vi "High_Voltage_Power_Supply_API.vi"(0 "COM Port In":refnum<visa-resource-name>, 2 "Control Mode (T = CV, F = CC)":bool=TRUE, 3 "CH1 ON/OFF (T = ON)":bool, 4 "CH2 ON/OFF (T = ON)":bool, 5 "MEASURE (T = measure)":bool, 6 "STOP (T = stop)":bool, 7 "error in (no error)":errorcluster, 10 "CH1 VOLTAGE SET (-2000...0 V)":i16 min=-2000 max=0 step=100, 11 "CH2 VOLTAGE SET (0...+2000 V)":i16 min=0 max=2000 step=100, 12 "CH1 CURRENT SET (0...5 mA)":dbl=5.0 min=0.0 max=5.0 step=0.1 format="%_4f", 13 "CH2 CURRENT SET (0...5 mA)":dbl=5.0 min=0.0 max=5.0 step=0.1 format="%_4f") -> (20 "COM Port Out":refnum<visa-resource-name>, 21 "Connection (T = active)":bool, 22 "Emergency Stop (T = active)":bool, 23 "CH1 VOLTAGE OUT (V)":i32, 24 "CH1 CURRENT OUT (mA)":dbl format="%#_4f", 25 "CH2 VOLTAGE OUT (V)":i32, 26 "CH2 CURRENT OUT (mA)":dbl format="%#_4f", 27 "error out":errorcluster)   [LabVIEW 2016]
doc: "This VI controls the High Voltage Power Supply.\n\nUsage: \n # Place this VI in a while loop for continuous operation\n\nExtra information:\n # 2 channels CH:\n * CH1 outputs -2000 to 0 V\n * CH2 outputs 0 to +2000 V\n * Both output 0 to 5 mA\n\n # Control Mode:\n * True = CV or Constant Voltage: \"VOLTAGE SET\" sets the output voltage \n and \"CURRENT SET\" sets the current limit\n * False = CC or Constant Current: \"CURRENT SET\" sets the output current \n and \"VOLTAGE SET\" sets the voltage limit\n\n # Connection (T = active)\n * Signals whether a connection is established\n\n # Emergency Stop (T = active)\n * Signals whether the emergency stop is on\n\n # Measure (T = measure):\n * True: Constant or pulse\n\n # Stop (T = stop)\n * True: Pulse\n * Resets the High Voltage Power Supply\n\nBachelor's thesis FIIW 3Ba EA-ICT 2017-2018:\n * Sven Baerten - sven.baerten@student.uhasselt.be\n * Wouter Falise - wouter.falise@student.uhasselt.be"
uses:
  High_Voltage_Power_Supply_API_States.ctl
  <vilib>/Instr/_visa.llb/VISA Configure Serial Port (Instr).vi
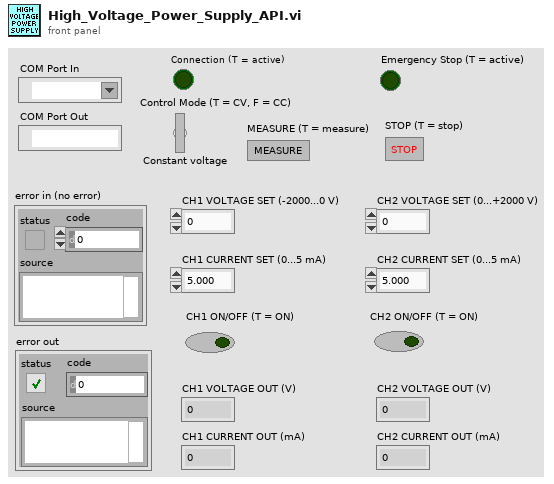
[diagram p1: front panel]
types:
  T1 = typedef "High_Voltage_Power_Supply_API_States.ctl" = enum16{"EMERGENCY_STOP", "NOT_SYNCHRONISED", "SYNCHRONISED"}
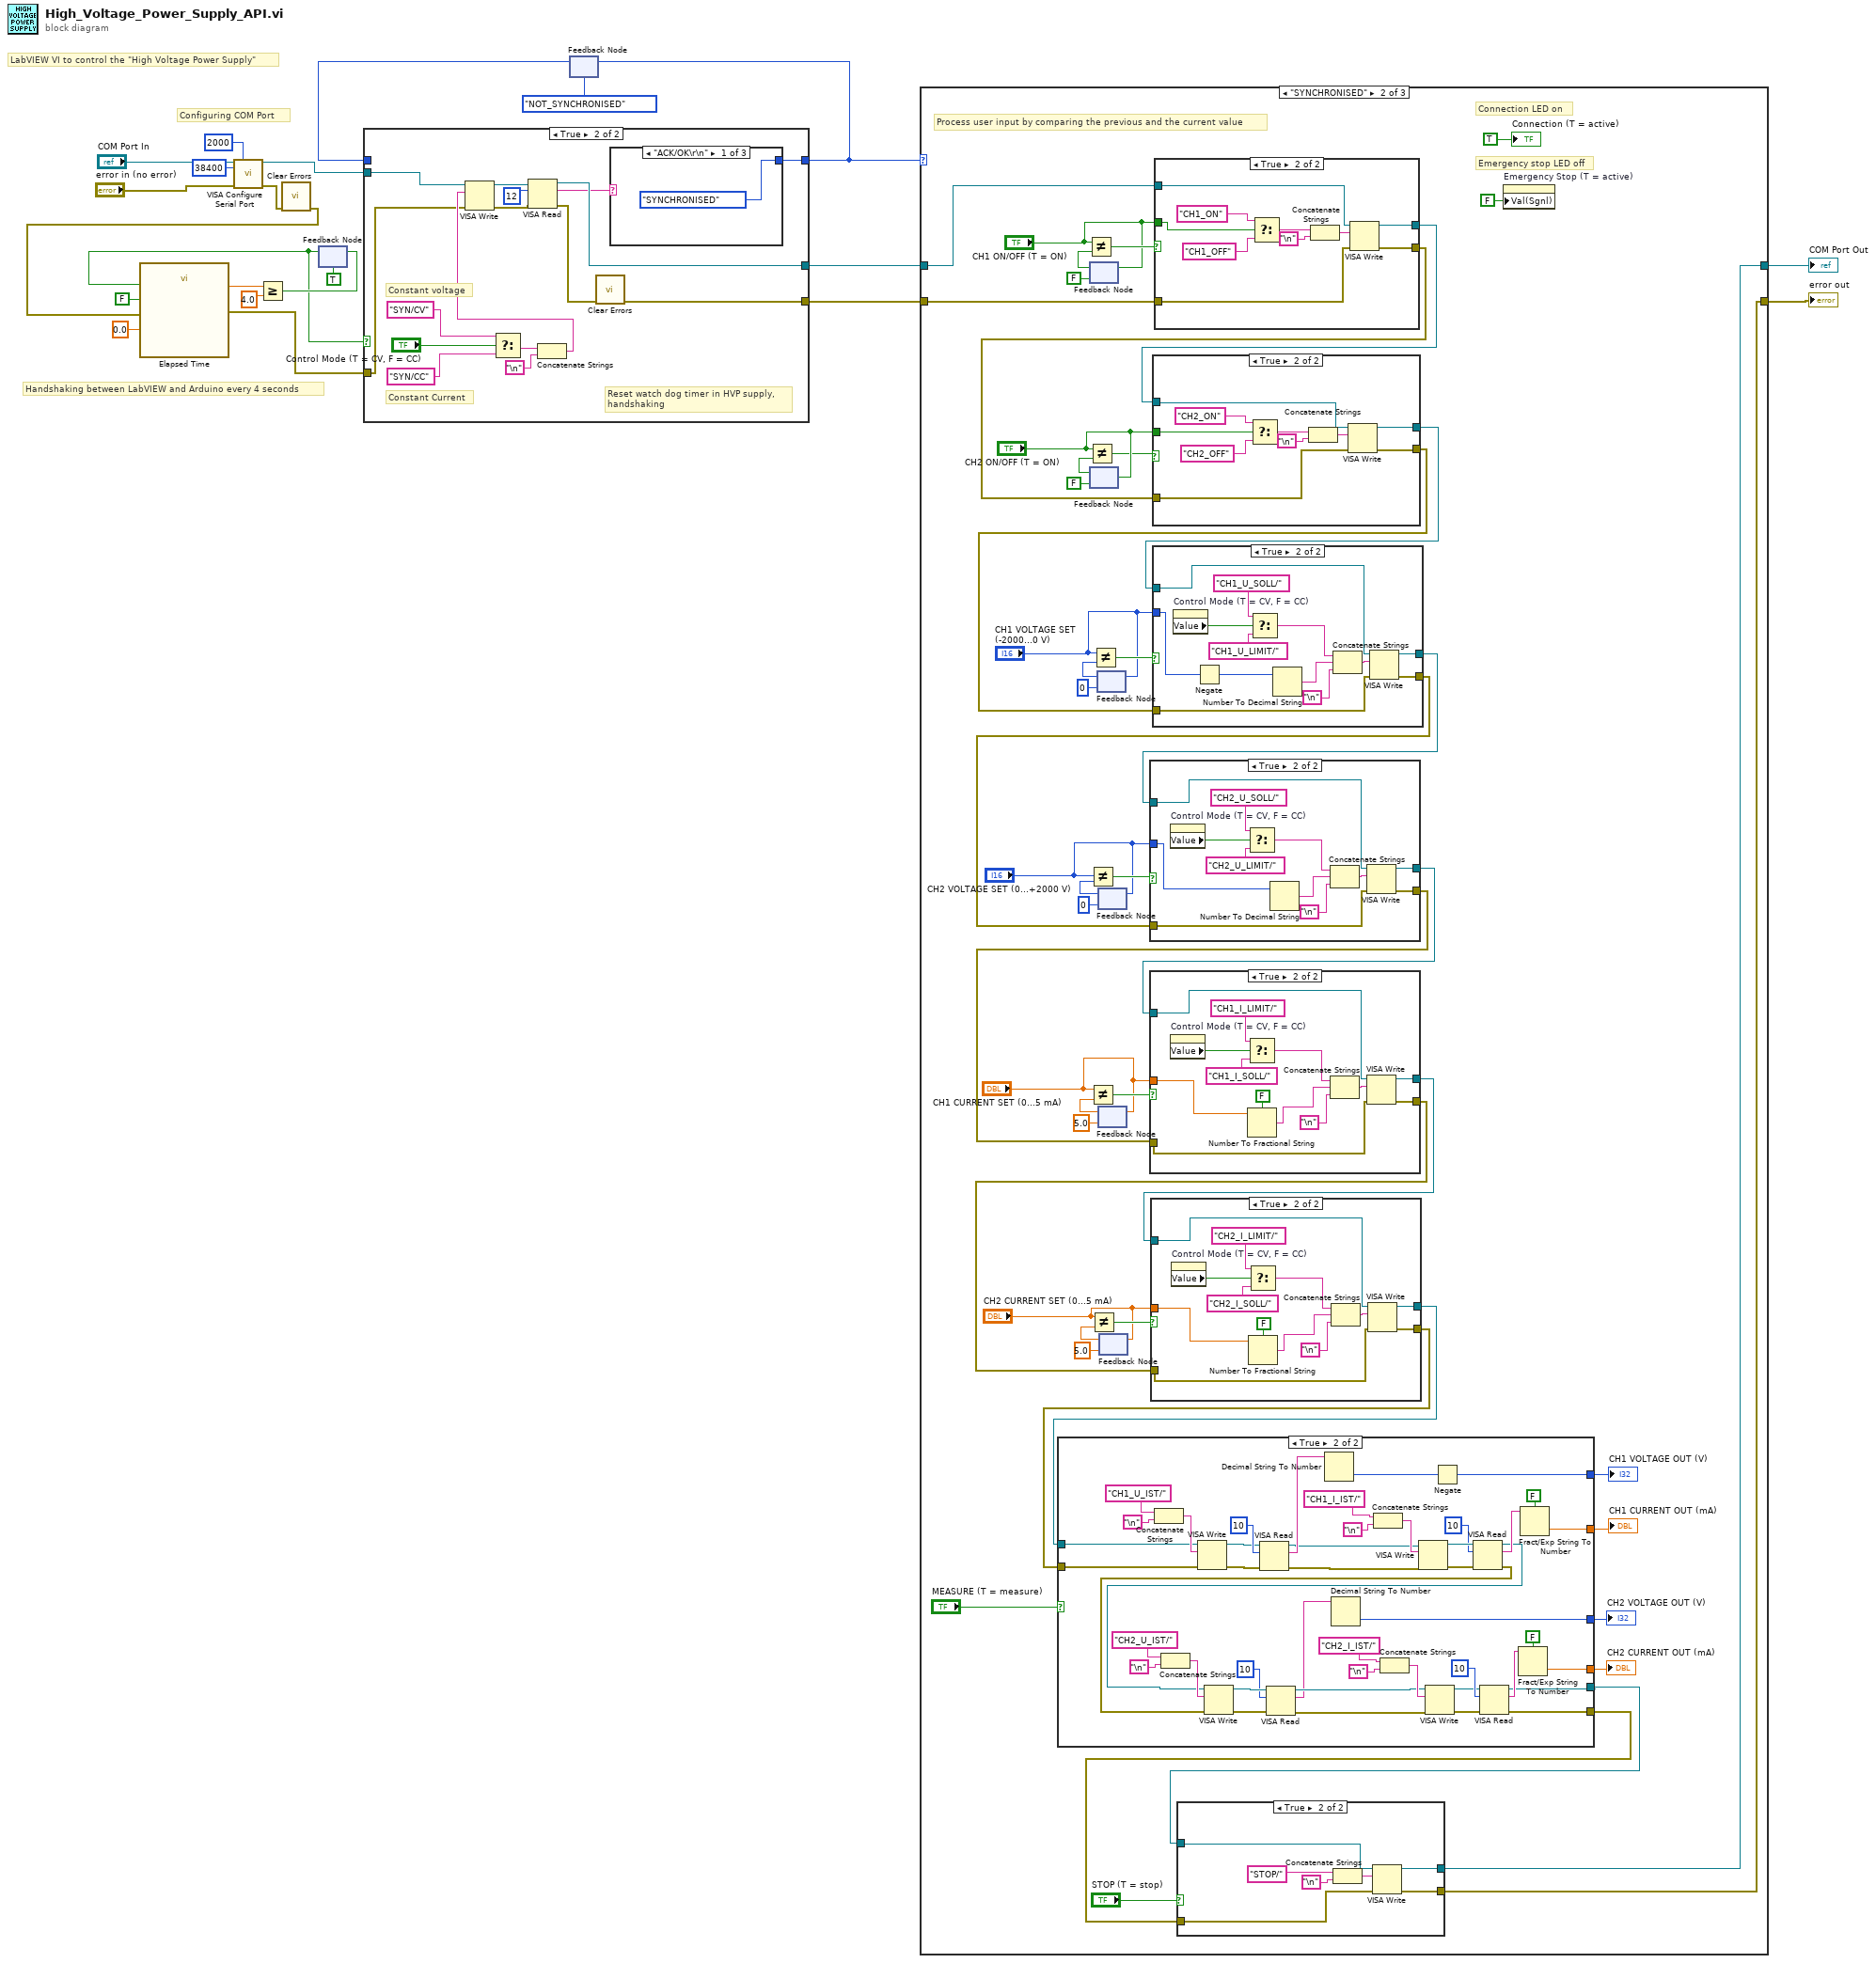
[diagram p0: block diagram]
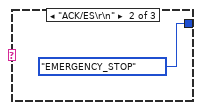
[diagram p3: hidden frame]
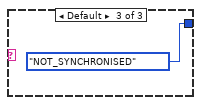
[diagram p4: hidden frame]
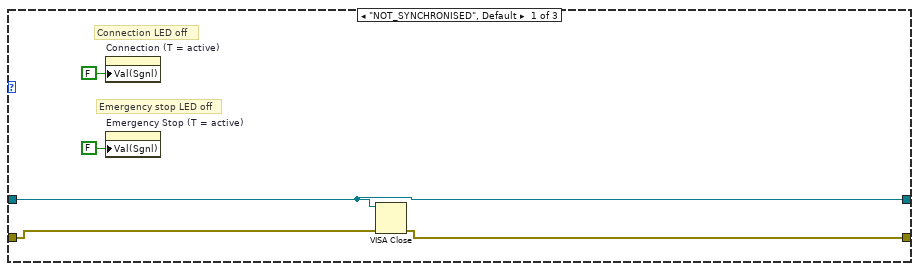
[diagram p5: hidden frame]
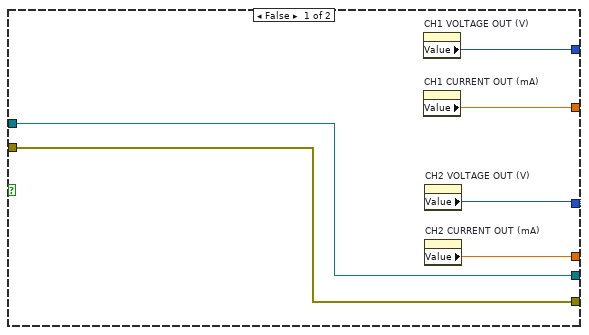
[diagram p7: hidden frame]
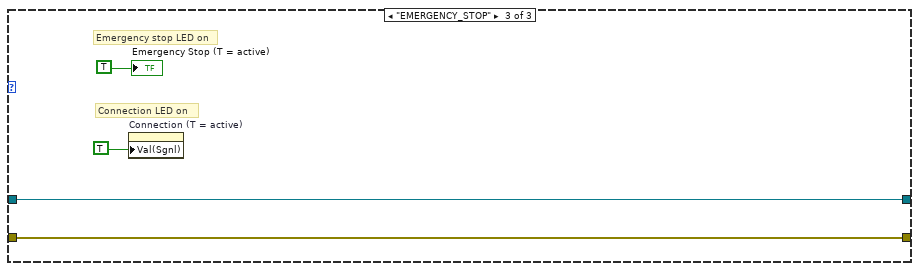
[diagram p14: hidden frame]
diagram:
  # "LabVIEW VI to control the \"High Voltage Power Supply\""
  # "Configuring COM Port"
  # "Handshaking between LabVIEW and Arduino every 4 seconds"
  n1 = call-poly "VISA Configure Serial Port"("VISA resource name"="COM Port In", "timeout (10sec)"=u32 2000, "baud rate (9600)"=u32 38400, "error in (no error)"="error in (no error)") -> ("VISA resource name out"=w7:refnum<visa-resource-name>, "error out"=w4:errorcluster)  [unwired: 10 in]
  n2 = call <vilib>:"Clear Errors.vi"("error in (no error)"=w4) -> ("error out"=w2:errorcluster)  [unwired: 5 in, 1 out]
  n3 = feedback #1(TRUE) -> (w8:bool)
  n4 = call "Elapsed Time"("Reset"=w8, "Auto Reset"=FALSE, "error in (no error)"=w2, "Set Start Time (s)"=0.0) -> ("Elapsed Time (s)"=w14:dbl, "error out"=w17:errorcluster)  [unwired: 8 in, 6 out]
  n5 = Greater Or Equal?(x=w14, y=4.0 ("Time Target (s)")) -> (x >= y?=w11:bool)
  n6 = feedback-in #1(w11) -> ()
  n7 = feedback #2(High_Voltage_Power_Supply_API_States."NOT_SYNCHRONISED") -> (w18:T1)
  n8 = case shown="True" w8 {
    tunnel: [w23 w28] -> w19
    tunnel: [w24 w26] -> w10
    tunnel: [w25 w29] -> w9
    tunnel: w7 -> [w25 w32]
    tunnel: w17 -> [w24 w31]
    tunnel: w18 -> [w23 _]
    frame False {
      # "No handshaking"
    }
    frame True {
      # "Constant voltage"
      # "Constant Current"
      # "Reset watch dog timer in HVP supply, \nhandshaking"
      n9 = Select(t="SYN/CV", s="Control Mode (T = CV, F = CC)", f="SYN/CC") -> (s? t:f=w39:string)
      n10 = Concatenate Strings(w39, "\n") -> (w38:string)
      n11 = VISA Write(VISA resource name=w32, write buffer=w38, error in (no error)=w31) -> (VISA resource name out=w37:refnum<visa-resource-name>, error out=w36:errorcluster)  [unwired: 1 out]
      n12 = VISA Read(VISA resource name=w37, byte count=u32 12, error in (no error)=w36) -> (VISA resource name out=w29:refnum<visa-resource-name>, read buffer=w27:string, error out=w30:errorcluster)  [unwired: 1 out]
      n13 = call <vilib>:"Clear Errors.vi"("error in (no error)"=w30) -> ("error out"=w26:errorcluster)  [unwired: 5 in, 1 out]
      n14 = case shown="\"ACK/OK\\r\\n\"" w27 {
        tunnel: [High_Voltage_Power_Supply_API_States."SYNCHRONISED" High_Voltage_Power_Supply_API_States."EMERGENCY_STOP" High_Voltage_Power_Supply_API_States."NOT_SYNCHRONISED"] -> w28
        frame "ACK/OK\r\n" {
        }
        frame "ACK/ES\r\n" {
        }
        frame Default {
        }
      }
    }
  }
  n15 = feedback-in #2(w19) -> ()
  n16 = case shown="\"SYNCHRONISED\"" w19 {
    tunnel: w10 -> [w47 w52 w245]
    tunnel: w9 -> [w46 w53 w244]
    tunnel: [w46 w57 w244] -> w22
    tunnel: [w45 w56 w245] -> w21
    frame "NOT_SYNCHRONISED", Default {
      # "Emergency stop LED off"
      # "Connection LED off"
      n17 = property on="Connection (T = active)" class="Bool (strict)"("Val(Sgnl)"=FALSE ("Value (Signaling)")) -> ()  [unwired: 2 in, 2 out]
      n18 = property on="Emergency Stop (T = active)" class="Bool (strict)"("Val(Sgnl)"=FALSE ("Value (Signaling)")) -> ()  [unwired: 2 in, 2 out]
      n19 = VISA Close(VISA resource name=w46, error in (no error)=w47) -> (error out=w45:errorcluster)
    }
    frame "SYNCHRONISED" {
      # "Emergency stop LED off"
      # "Connection LED on"
      # "Process user input by comparing the previous and the current value"
      n20 = feedback-in #3("CH1 ON/OFF (T = ON)") -> ()
      n21 = feedback #3(FALSE ("CH1 ON/OFF (T = ON)")) -> (w99:bool)
      n22 = Not Equal?(x="CH1 ON/OFF (T = ON)", y=w99) -> (x != y?=w98:bool)
      n23 = feedback #4(FALSE ("CH2 ON/OFF (T = ON)")) -> (w96:bool)
      n24 = Not Equal?(x="CH2 ON/OFF (T = ON)", y=w96) -> (x != y?=w94:bool)
      n25 = feedback-in #4("CH2 ON/OFF (T = ON)") -> ()
      n26 = feedback #5(i16 0 ("CH1 VOLTAGE")) -> (w91:i16)
      n27 = Not Equal?(x="CH1 VOLTAGE SET (-2000...0 V)", y=w91) -> (x != y?=w90:bool)
      n28 = feedback-in #5("CH1 VOLTAGE SET (-2000...0 V)") -> ()
      n29 = feedback #6(i16 0 ("CH2 VOLTAGE")) -> (w85:i16)
      n30 = Not Equal?(x="CH2 VOLTAGE SET (0...+2000 V)", y=w85) -> (x != y?=w86:bool)
      n31 = feedback-in #6("CH2 VOLTAGE SET (0...+2000 V)") -> ()
      n32 = feedback #7(5.0 ("CH1 CURRENT")) -> (w82:dbl)
      n33 = Not Equal?(x="CH1 CURRENT SET (0...5 mA)", y=w82) -> (x != y?=w81:bool)
      n34 = feedback-in #7("CH1 CURRENT SET (0...5 mA)") -> ()
      n35 = feedback #8(5.0 ("CH2 CURRENT")) -> (w75:dbl)
      n36 = Not Equal?(x="CH2 CURRENT SET (0...5 mA)", y=w75) -> (x != y?=w76:bool)
      n37 = feedback-in #8("CH2 CURRENT SET (0...5 mA)") -> ()
      n38 = case shown="True" w98 {
        tunnel: "CH1 ON/OFF (T = ON)" -> [_ w237]
        tunnel: [w231 w236] -> w93
        tunnel: [w232 w235] -> w92
        tunnel: w53 -> [w232 w234]
        tunnel: w52 -> [w231 w233]
        frame False {
        }
        frame True {
          n39 = Select(t="CH1_ON", s=w237, f="CH1_OFF") -> (s? t:f=w242:string)
          n40 = Concatenate Strings(w242, "\n") -> (w239:string)
          n41 = VISA Write(VISA resource name=w234, write buffer=w239, error in (no error)=w233) -> (VISA resource name out=w235:refnum<visa-resource-name>, error out=w236:errorcluster)  [unwired: 1 out]
        }
      }
      n42 = case shown="True" w94 {
        tunnel: "CH2 ON/OFF (T = ON)" -> [_ w225]
        tunnel: w92 -> [w219 w224]
        tunnel: w93 -> [w220 w223]
        tunnel: [w220 w222] -> w87
        tunnel: [w219 w221] -> w88
        frame False {
        }
        frame True {
          n43 = Select(t="CH2_ON", s=w225, f="CH2_OFF") -> (s? t:f=w230:string)
          n44 = Concatenate Strings(w230, "\n") -> (w227:string)
          n45 = VISA Write(VISA resource name=w224, write buffer=w227, error in (no error)=w223) -> (VISA resource name out=w221:refnum<visa-resource-name>, error out=w222:errorcluster)  [unwired: 1 out]
        }
      }
      n46 = case shown="True" w90 {
        tunnel: "CH1 VOLTAGE SET (-2000...0 V)" -> [_ w207]
        tunnel: w88 -> [w205 w211]
        tunnel: w87 -> [w204 w210]
        tunnel: [w205 w209] -> w83
        tunnel: [w204 w208] -> w84
        frame False {
        }
        frame True {
          n47 = property on="Control Mode (T = CV, F = CC)" class="Bool (strict)"() -> ("Value"=w216:bool)  [unwired: 2 in, 2 out]
          n48 = Negate(x=w207) -> (-x=w206:i16)
          n49 = Select(t="CH1_U_SOLL/", s=w216, f="CH1_U_LIMIT/") -> (s? t:f=w213:string)
          n50 = Number To Decimal String(number=w206) -> (decimal integer string=w217:string)  [unwired: 1 in]
          n51 = Concatenate Strings(w213, w217, "\n") -> (w218:string)
          n52 = VISA Write(VISA resource name=w211, write buffer=w218, error in (no error)=w210) -> (VISA resource name out=w209:refnum<visa-resource-name>, error out=w208:errorcluster)  [unwired: 1 out]
        }
      }
      n53 = case shown="True" w86 {
        tunnel: w83 -> [w191 w196]
        tunnel: w84 -> [w190 w195]
        tunnel: [w191 w194] -> w79
        tunnel: [w190 w193] -> w80
        tunnel: "CH2 VOLTAGE SET (0...+2000 V)" -> [_ w192]
        frame False {
        }
        frame True {
          n54 = property on="Control Mode (T = CV, F = CC)" class="Bool (strict)"() -> ("Value"=w201:bool)  [unwired: 2 in, 2 out]
          n55 = Select(t="CH2_U_SOLL/", s=w201, f="CH2_U_LIMIT/") -> (s? t:f=w198:string)
          n56 = Number To Decimal String(number=w192) -> (decimal integer string=w202:string)  [unwired: 1 in]
          n57 = Concatenate Strings(w198, w202, "\n") -> (w203:string)
          n58 = VISA Write(VISA resource name=w196, write buffer=w203, error in (no error)=w195) -> (VISA resource name out=w194:refnum<visa-resource-name>, error out=w193:errorcluster)  [unwired: 1 out]
        }
      }
      n59 = case shown="True" w81 {
        tunnel: w79 -> [w176 w183]
        tunnel: w80 -> [w175 w182]
        tunnel: [w176 w181] -> w73
        tunnel: [w175 w180] -> w74
        tunnel: "CH1 CURRENT SET (0...5 mA)" -> [_ w177]
        frame False {
        }
        frame True {
          n60 = property on="Control Mode (T = CV, F = CC)" class="Bool (strict)"() -> ("Value"=w188:bool)  [unwired: 2 in, 2 out]
          n61 = Select(t="CH1_I_LIMIT/", s=w188, f="CH1_I_SOLL/") -> (s? t:f=w185:string)
          n62 = Number To Fractional String(use system decimal point (T)=FALSE, number=w177) -> (F-format string=w178:string)  [unwired: 2 in]
          n63 = Concatenate Strings(w185, w178, "\n") -> (w189:string)
          n64 = VISA Write(VISA resource name=w183, write buffer=w189, error in (no error)=w182) -> (VISA resource name out=w181:refnum<visa-resource-name>, error out=w180:errorcluster)  [unwired: 1 out]
        }
      }
      n65 = case shown="True" w76 {
        tunnel: w73 -> [w161 w168]
        tunnel: w74 -> [w160 w167]
        tunnel: [w161 w166] -> w70
        tunnel: [w160 w165] -> w71
        tunnel: "CH2 CURRENT SET (0...5 mA)" -> [_ w162]
        frame False {
        }
        frame True {
          n66 = property on="Control Mode (T = CV, F = CC)" class="Bool (strict)"() -> ("Value"=w173:bool)  [unwired: 2 in, 2 out]
          n67 = Select(t="CH2_I_LIMIT/", s=w173, f="CH2_I_SOLL/") -> (s? t:f=w170:string)
          n68 = Number To Fractional String(use system decimal point (T)=FALSE, number=w162) -> (F-format string=w163:string)  [unwired: 2 in]
          n69 = Concatenate Strings(w170, w163, "\n") -> (w174:string)
          n70 = VISA Write(VISA resource name=w168, write buffer=w174, error in (no error)=w167) -> (VISA resource name out=w166:refnum<visa-resource-name>, error out=w165:errorcluster)  [unwired: 1 out]
        }
      }
      n71 = case shown="True" "MEASURE (T = measure)" {
        tunnel: w70 -> [w114 w122]
        tunnel: [w114 w127] -> w55
        tunnel: w71 -> [w113 w121]
        tunnel: [w113 w126] -> w54
        tunnel: [w111 w116] -> w68
        tunnel: [w112 w125] -> w67
        tunnel: [w109 w124] -> w66
        tunnel: [w110 w123] -> w65
        frame False {
          n72 = property on="CH1 VOLTAGE OUT (V)" class="DigNum (strict)"() -> ("Value"=w111:i32)  [unwired: 2 in, 2 out]
          n73 = property on="CH1 CURRENT OUT (mA)" class="DigNum (strict)"() -> ("Value"=w112:dbl)  [unwired: 2 in, 2 out]
          n74 = property on="CH2 VOLTAGE OUT (V)" class="DigNum (strict)"() -> ("Value"=w109:i32)  [unwired: 2 in, 2 out]
          n75 = property on="CH2 CURRENT OUT (mA)" class="DigNum (strict)"() -> ("Value"=w110:dbl)  [unwired: 2 in, 2 out]
        }
        frame True {
          n76 = Concatenate Strings("CH1_U_IST/", "\n") -> (w147:string)
          n77 = Concatenate Strings("CH2_U_IST/", "\n") -> (w144:string)
          n78 = VISA Write(VISA resource name=w122, write buffer=w147, error in (no error)=w121) -> (VISA resource name out=w149:refnum<visa-resource-name>, error out=w150:errorcluster)  [unwired: 1 out]
          n79 = VISA Read(VISA resource name=w149, byte count=u32 10, error in (no error)=w150) -> (VISA resource name out=w120:refnum<visa-resource-name>, read buffer=w152:string, error out=w119:errorcluster)  [unwired: 1 out]
          n80 = Decimal String To Number(string=w152) -> (number=w115:i32)  [unwired: 2 in, 1 out]
          n81 = Concatenate Strings("CH1_I_IST/", "\n") -> (w157:string)
          n82 = Concatenate Strings("CH2_I_IST/", "\n") -> (w135:string)
          n83 = VISA Write(VISA resource name=w120, write buffer=w157, error in (no error)=w119) -> (VISA resource name out=w155:refnum<visa-resource-name>, error out=w154:errorcluster)  [unwired: 1 out]
          n84 = Negate(x=w115) -> (-x=w116:i32)
          n85 = VISA Read(VISA resource name=w155, byte count=u32 10, error in (no error)=w154) -> (VISA resource name out=w129:refnum<visa-resource-name>, read buffer=w159:string, error out=w128:errorcluster)  [unwired: 1 out]
          n86 = VISA Write(VISA resource name=w129, write buffer=w144, error in (no error)=w128) -> (VISA resource name out=w142:refnum<visa-resource-name>, error out=w141:errorcluster)  [unwired: 1 out]
          n87 = VISA Read(VISA resource name=w142, byte count=u32 10, error in (no error)=w141) -> (VISA resource name out=w132:refnum<visa-resource-name>, read buffer=w130:string, error out=w131:errorcluster)  [unwired: 1 out]
          n88 = Decimal String To Number(string=w130) -> (number=w124:i32)  [unwired: 2 in, 1 out]
          n89 = VISA Write(VISA resource name=w132, write buffer=w135, error in (no error)=w131) -> (VISA resource name out=w137:refnum<visa-resource-name>, error out=w138:errorcluster)  [unwired: 1 out]
          n90 = VISA Read(VISA resource name=w137, byte count=u32 10, error in (no error)=w138) -> (VISA resource name out=w127:refnum<visa-resource-name>, read buffer=w133:string, error out=w126:errorcluster)  [unwired: 1 out]
          n91 = Fract/Exp String To Number(use system decimal point (T)=FALSE, string=w133) -> (number=w123:dbl)  [unwired: 2 in, 1 out]
          n92 = Fract/Exp String To Number(use system decimal point (T)=FALSE, string=w159) -> (number=w125:dbl)  [unwired: 2 in, 1 out]
        }
      }
      "CH1 VOLTAGE OUT (V)" <- w68
      "CH1 CURRENT OUT (mA)" <- w67
      "CH2 VOLTAGE OUT (V)" <- w66
      "CH2 CURRENT OUT (mA)" <- w65
      n93 = case shown="True" "STOP (T = stop)" {
        tunnel: w55 -> [w100 w106]
        tunnel: w54 -> [w101 w105]
        tunnel: [w101 w104] -> w56
        tunnel: [w100 w103] -> w57
        frame False {
        }
        frame True {
          n94 = Concatenate Strings("STOP/" ("string"), "\n") -> (w108:string)
          n95 = VISA Write(VISA resource name=w106, write buffer=w108, error in (no error)=w105) -> (VISA resource name out=w103:refnum<visa-resource-name>, error out=w104:errorcluster)  [unwired: 1 out]
        }
      }
      n96 = property on="Emergency Stop (T = active)" class="Bool (strict)"("Val(Sgnl)"=FALSE ("Value (Signaling)")) -> ()  [unwired: 2 in, 2 out]
      "Connection (T = active)" <- TRUE ("Connection")
    }
    frame "EMERGENCY_STOP" {
      # "Connection LED on"
      # "Emergency stop LED on"
      n97 = property on="Connection (T = active)" class="Bool (strict)"("Val(Sgnl)"=TRUE ("Value (Signaling)")) -> ()  [unwired: 2 in, 2 out]
      "Emergency Stop (T = active)" <- TRUE ("Emergency Stop")
    }
  }
  "error out" <- w21
  "COM Port Out" <- w22
